vi "Create Cursor.vi"(8 "error in (no error)":errorcluster, 10 "SQLite3LV Connection":refnum<class "sqlite3.lvclass">) -> (0 "error out":errorcluster, 3 "SQLite3LV Cursor out":refnum<class "cursor.lvclass">)   [LabVIEW 2014, in "SQLite3LV.lvlib" / "cursor.lvclass"]
uses:
  cursor.lvclass
  SQLite3 Class/sqlite3.lvclass
  ctl_active_statement.ctl
  cursor.lvclass/cursor.ctl
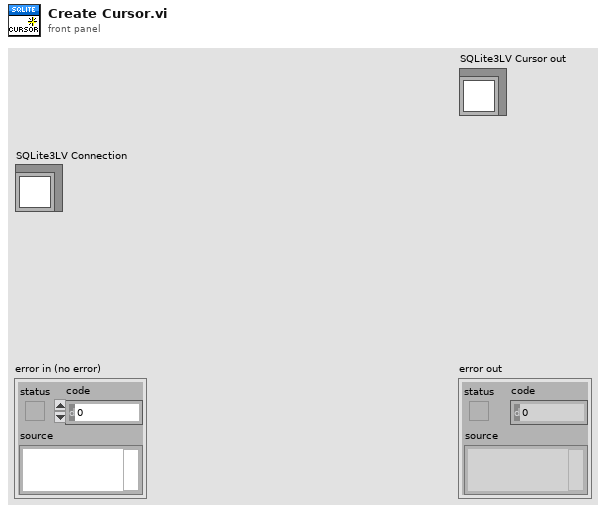
[diagram p1: front panel]
types:
  T1 = typedef "SQLite3LV.lvlib/cursor.lvclass/ctl_active_statement.ctl" = cluster{"ppStmt":i64, "column count":i32, "bind offset":i32, "bind param count":i32, "finished?":bool, "column offset":i32, "column types":i32[]}
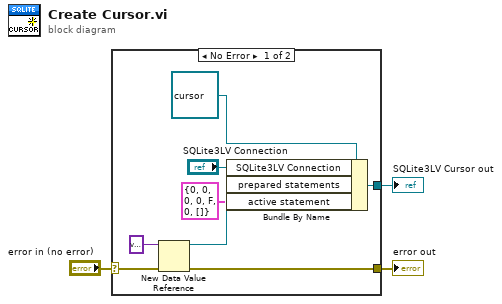
[diagram p0: block diagram]
diagram:
  n1 = case shown="No Error" "error in (no error)" {
    selector: "error in (no error)" -> [w6 w12]
    tunnel: [w4 w12] -> w2
    tunnel: [w10 _] -> w1
    frame No Error {
      n2 = New Data Value Reference(data value=variant ("variant"), error in=w6) -> (data value reference=w7:refnum<data-value>, error out=w4:errorcluster)
      n3 = Bundle By Name(cluster=refnum<class "cursor.lvclass"> refnum ("cursor in"), "SQLite3LV Connection"="SQLite3LV Connection", "prepared statements"=w7, "active statement"=T1 {"ppStmt"=0, "column count"=0, "bind offset"=0, "bind param count"=0, "finished?"=FALSE, "column offset"=0, "column types"=[]}) -> (w10:refnum<class "cursor.lvclass">)
    }
    frame Error {
    }
  }
  "error out" <- w2
  "SQLite3LV Cursor out" <- w1
